vi "draw_desired_heading.vi"(6 "circle color":u32(colorbox)=16746026, 8 "Length of line (px)":dbl=50.0 format="%#_13g", 9 "Boat Position":cluster{"X":i32, "Y":i32}, 10 "Desired Heading":dbl format="%#_13g", 11 "Image In":T1) -> (3 "Image Out":T1)   [LabVIEW 2013]
doc: "Places al line on the map for the desired heading\n\nEric Schneider, July 2014"
uses:
  <vilib>/vision/Image Controls.llb/IMAQ Image.ctl
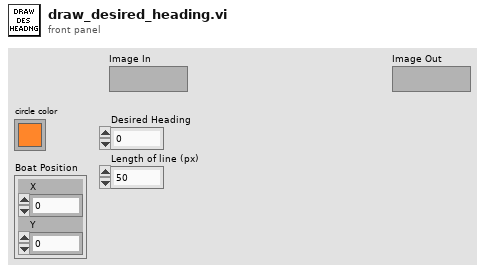
[diagram p1: front panel]
types:
  T1 = typedef "IMAQ Image.ctl" = refnum<image>
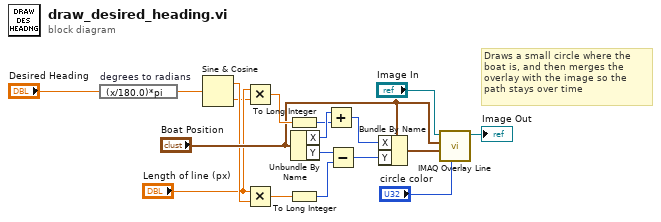
[diagram p0: block diagram]
diagram:
  # "Draws a small circle where the boat is, and then merges the overlay with the image so the path stays over time"
  n1 = expression code="(x/180.0)*pi" "degrees to radians"("Desired Heading") -> (w9:dbl)
  n2 = Sine & Cosine(0:w9) -> (1:w8:dbl, 2:w6:dbl)
  n3 = Multiply(x="Length of line (px)", y=w6) -> (x*y=w13:dbl)
  n4 = Multiply(x="Length of line (px)", y=w8) -> (x*y=w5:dbl)
  n5 = To Long Integer(number=w13) -> (32bit integer=w12:i32)
  n6 = To Long Integer(number=w5) -> (32bit integer=w2:i32)
  n7 = Unbundle By Name("Boat Position") -> ("X"=w15:i32, "Y"=w3:i32)
  n8 = Add(x=w15, y=w12) -> (x+y=w10:i32)
  n9 = Subtract(x=w3, y=w2) -> (x-y=w1:i32)
  n10 = Bundle By Name(cluster="Boat Position", "X"=w10, "Y"=w1) -> (w4:cluster{"X":i32, "Y":i32})
  n11 = call "IMAQ Overlay Line"("Color"="circle color", "End Point"=w4, "Start Point"="Boat Position", "Image"="Image In") -> ("Image Out"=→"Image Out":T1)  [unwired: 6 in, 1 out]
